vi "load_xml.vi"(8 "error in":errorcluster, 10 "child node in":refnum<k20>, 11 "DAQmx_pulse_out (in)":refnum<class "DAQmx_DO.lvclass">) -> (0 "error out":errorcluster, 2 "child node out":refnum<k20>, 3 "DAQmx_pulse_out":refnum<class "DAQmx_DO.lvclass">)   [LabVIEW 2014, in "DAQmx_DO.lvclass"]
doc: "Loads DAQmx pulse output settings from xml. Expected format:\n\n<EnableDAQmxPulses>%b</EnableDAQmxPulses>\n<ResourceName>%s</ResourceName>\n<ClockRate>%f</ClockRate>\n<unitsPerSecond>%f</unitsPerSecond>\n<StartTrigger.WaitForStartTrigger>%b</StartTrigger.WaitForStartTrigger>\n<StartTrigger.source>%s</StartTrigger.source>\n<StartTrigger.edge>%s</StartTrigger.edge>\n<TimingSequenceControl columns=\"Description, Active?, Idle State,Off 0,On 0,Off 1,On 1,etc.\">\n<channel>%s</channel>\n</TimingSequenceControl>\n\nMTL 2013 Jan 1"
uses:
  DAQmx_DO.lvclass
  DAQmx_DO.lvclass/DAQmx_DO.ctl
  Globals.vi
  <vilib>/xml/Close Reference(Node).vi
  <resource>/objmgr/DOMUserDefRef.rc
  <vilib>/xml/NI_XML.lvlib
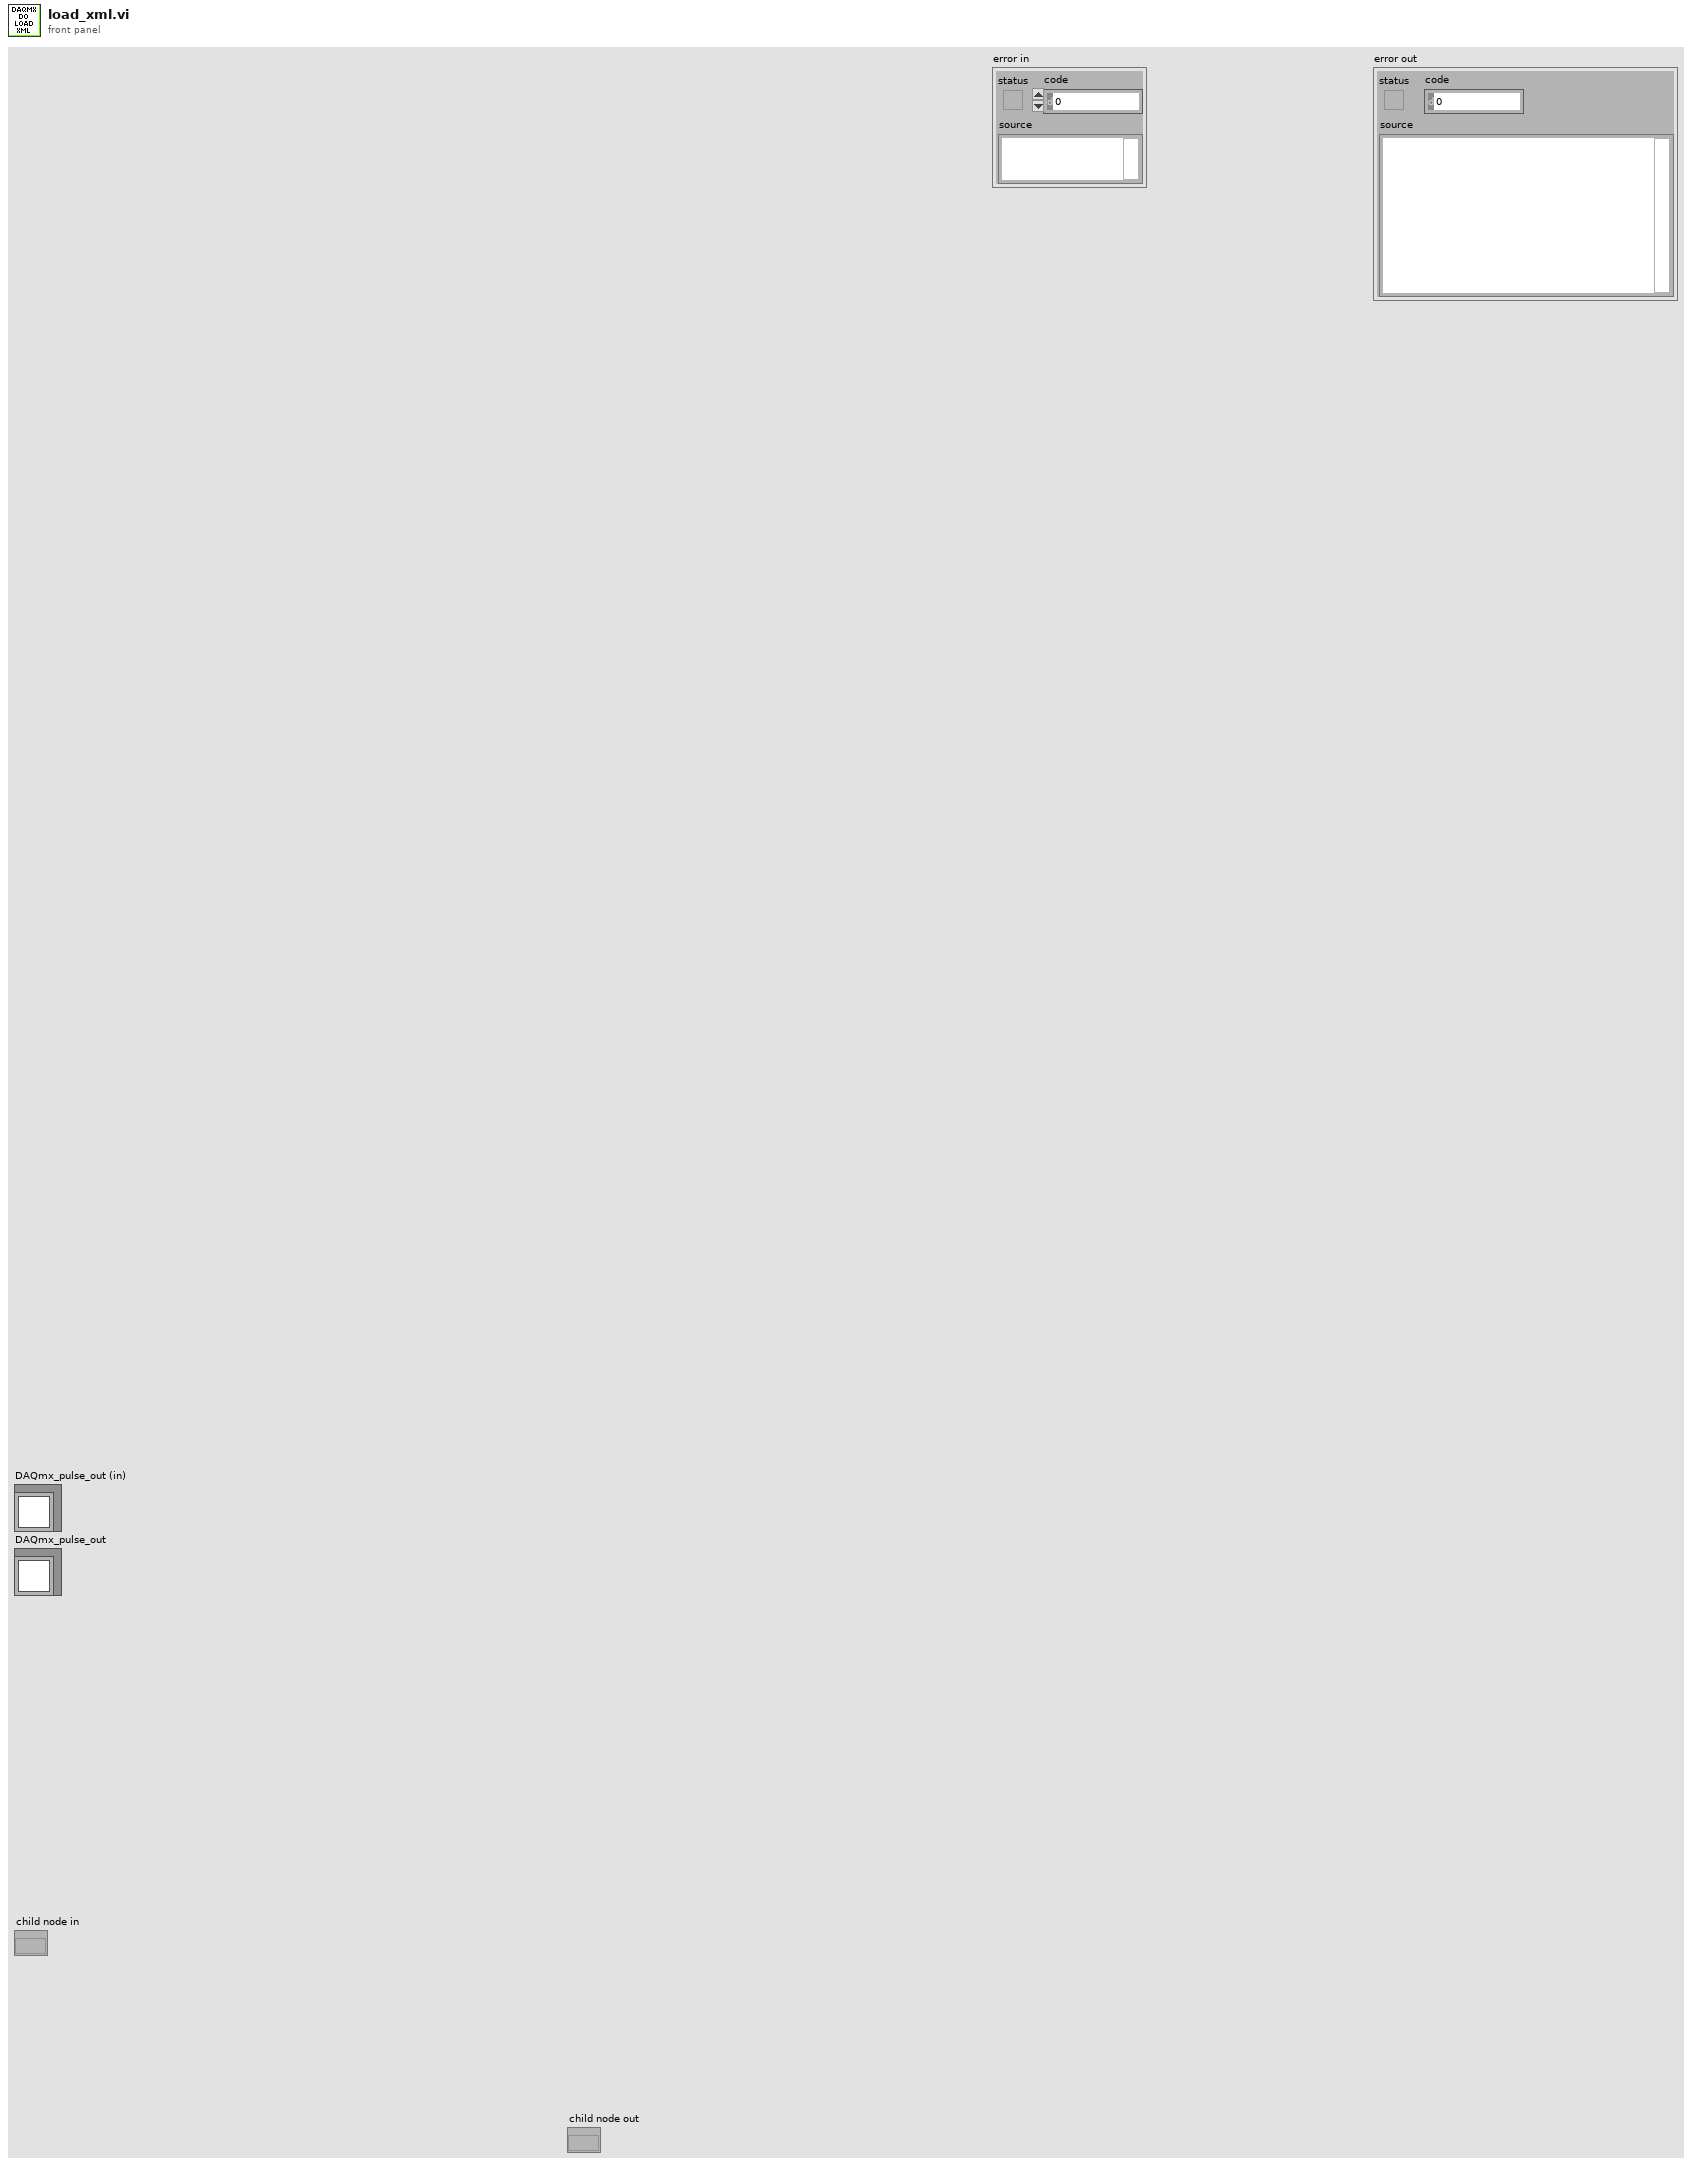
[diagram p1: front panel]
types:
  T1 = typedef "DAQmx_DO.lvclass/settings.ctl" = cluster{"Enable DAQmx Pulses":bool, "DAQmx Physical Channels":tag, "Clock Rate":dbl, "units/sec (ms=1000)":dbl, "Start Trigger":cluster{"Wait for start trigger?":bool, "source":tag, "edge":i32}, "waveform":T2}
  T2 = typedef "HSDIO.lvclass/waveform.ctl" = cluster{"name":string, "transitions":u32[], "states":u8[][]}
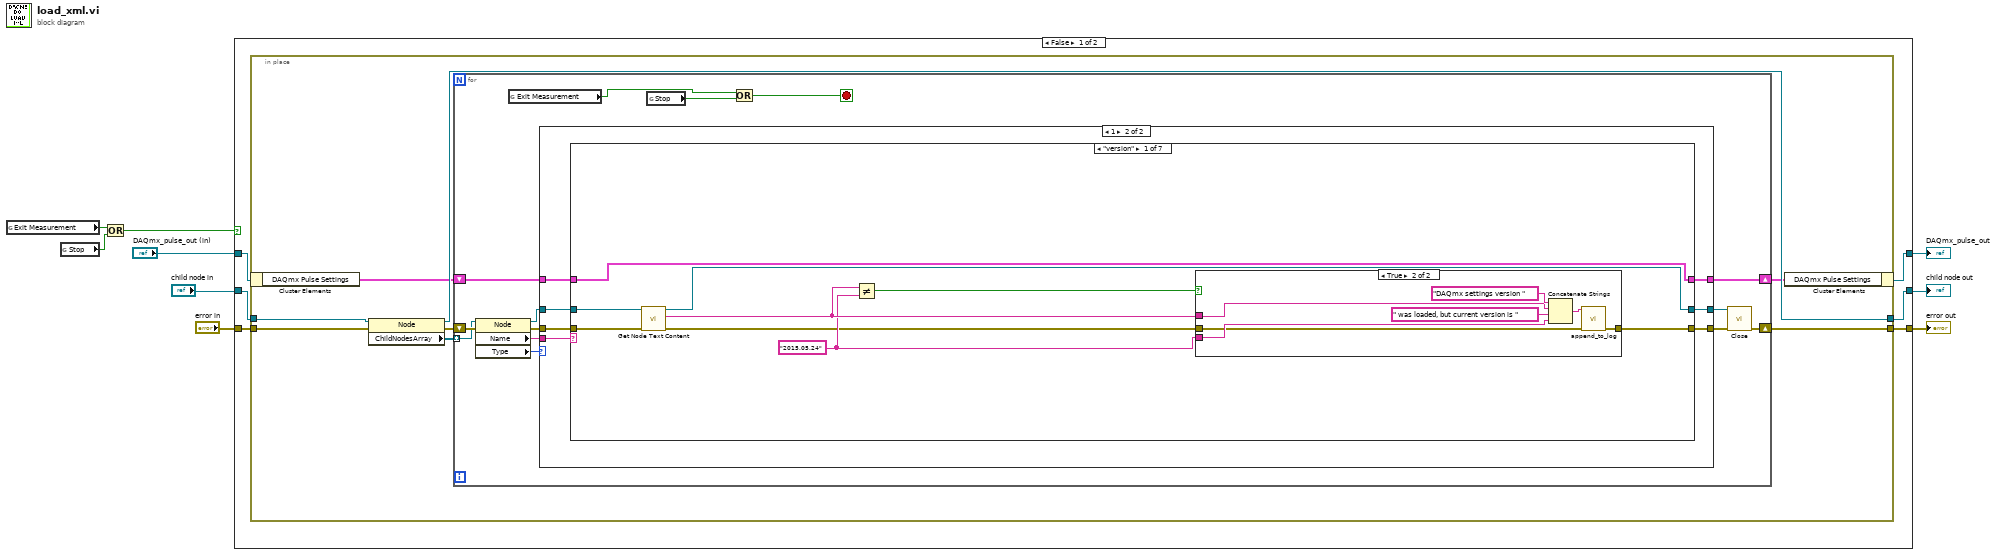
[diagram p0: block diagram]
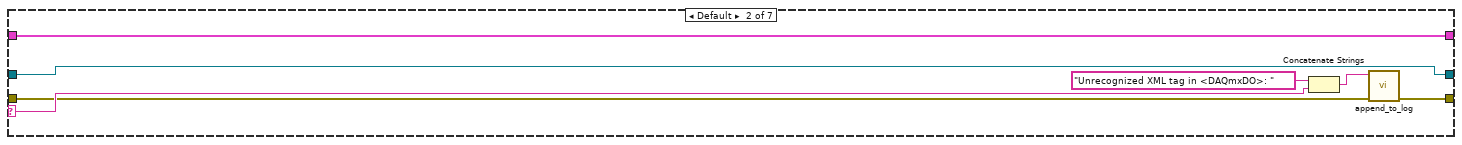
[diagram p4: hidden frame]
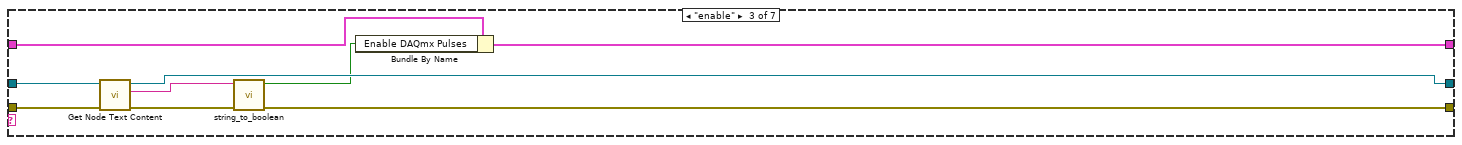
[diagram p5: hidden frame]
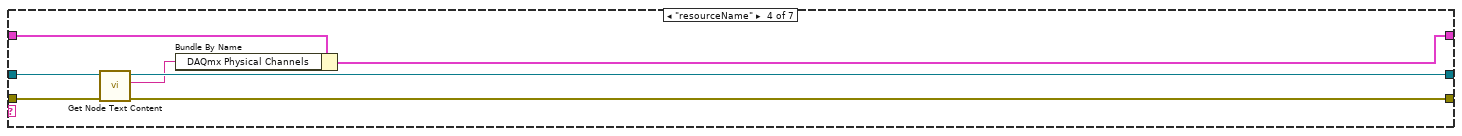
[diagram p6: hidden frame]
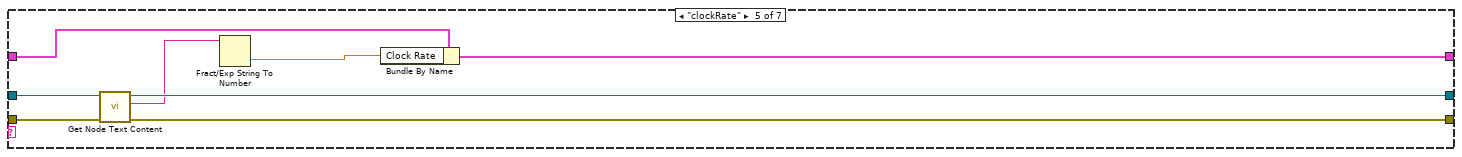
[diagram p7: hidden frame]
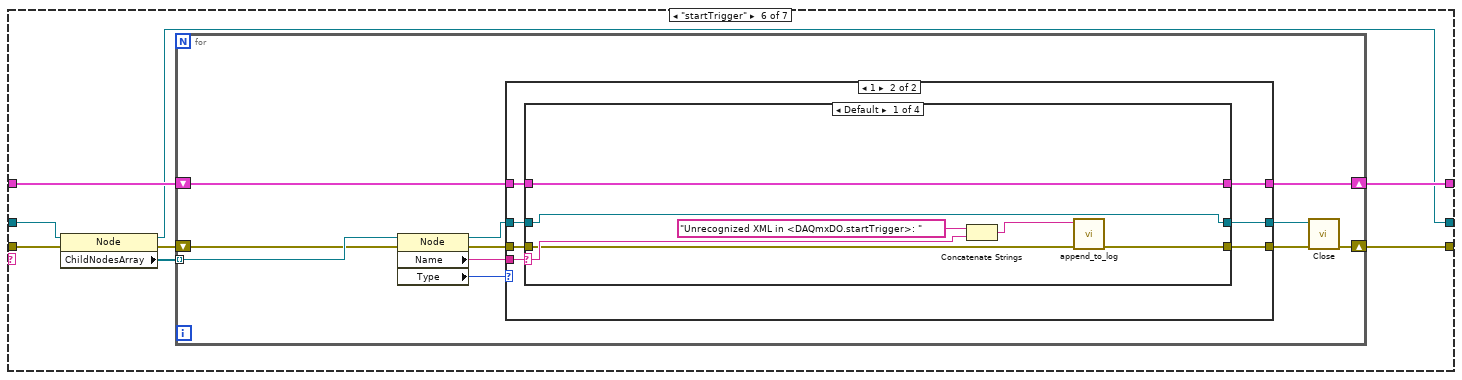
[diagram p8: hidden frame]
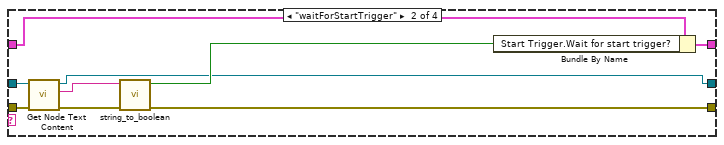
[diagram p10: hidden frame]
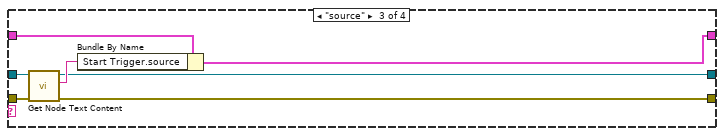
[diagram p11: hidden frame]
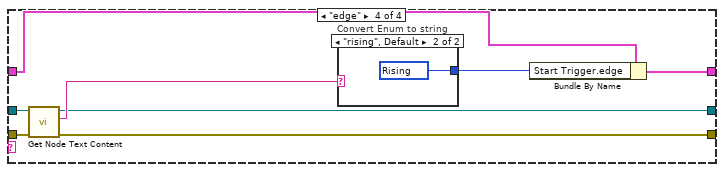
[diagram p12: hidden frame]
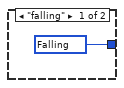
[diagram p13: hidden frame]
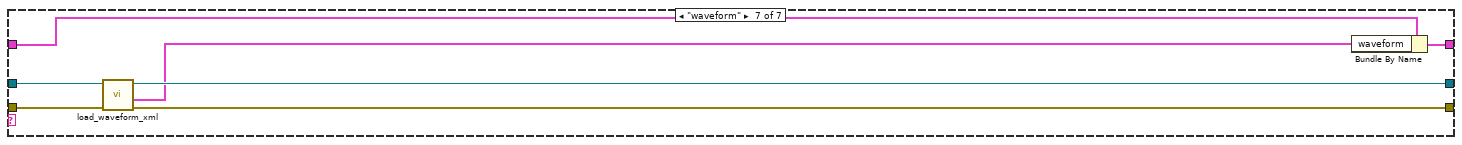
[diagram p14: hidden frame]
diagram:
  n1 = global read "Globals.vi" "Exit Measurement"() -> (w8:bool)
  n2 = global read "Globals.vi" "Stop"() -> (w9:bool)
  n3 = Or(x=w8, y=w9) -> (x .or. y?=w7:bool)
  n4 = case shown="False" w7 {
    tunnel: "DAQmx_pulse_out (in)" -> [w15 w167]
    tunnel: [w14 w167] -> w5
    tunnel: "error in" -> [w13 w166]
    tunnel: [w12 w166] -> w3
    tunnel: "child node in" -> [w11 w165]
    tunnel: [w10 w165] -> w1
    frame False {
      n5 = in-place {
        in-place-border: w13 -> [w21]
        in-place-border: [w20] -> w12
        in-place-border: w11 -> [w19]
        in-place-border: [w18] -> w10
        n6 = in-place-cluster #1(w15) -> ("DAQmx Pulse Settings"=w17:T1)
        n7 = property class="Node"(reference=w19, error in=w21) -> (reference out=w18:refnum<k20>, error out=w22:errorcluster, "ChildNodesArray"=w23:refnum<k20>[])
        n8 = for {
          tunnel: w23 -> [w28] mode=indexing
          shift-right: [w34] -> w16
          shift-left: w17 -> [w35]
          shift-right: [w31] -> w20
          shift-left: w22 -> [w29]
          stop <- w25 stop-if-true
          n9 = property class="Node"(reference=w28, error in=w29) -> (reference out=w36:refnum<k20>, error out=w32:errorcluster, "Name"=w37:string, "Type"=w24:i32)
          n10 = global read "Globals.vi" "Exit Measurement"() -> (w26:bool)
          n11 = case shown="1" w24 {
            tunnel: w37 -> [_ w47]
            tunnel: w36 -> [w39 w46]
            tunnel: w35 -> [w38 w45]
            tunnel: [w38 w44] -> w34
            tunnel: [w39 w43] -> w33
            tunnel: w32 -> [w40 w42]
            tunnel: [w40 w41] -> w30
            frame 0, Default {
            }
            frame 1 {
              n12 = case shown="\"version\"" w47 {
                selector: w47 -> [_ w67 _ _ _ _ _]
                tunnel: w46 -> [w51 w70 w79 w84 w92 w100 w162]
                tunnel: w45 -> [w49 w71 w77 w87 w95 w99 w164]
                tunnel: [w49 w71 w76 w86 w94 w97 w163] -> w44
                tunnel: [w50 w70 w80 w85 w93 w96 w161] -> w43
                tunnel: w42 -> [w52 w66 w78 w83 w91 w101 w159]
                tunnel: [w48 w65 w72 w82 w90 w98 w160] -> w41
                frame "version" {
                  w54 = "2015.05.24" ("y")
                  n13 = call <vilib>:"Get Node Text Content.vi"("error in (no error)"=w52, "node in"=w51) -> ("error out"=w53:errorcluster, "node text"=w55:string, "node out"=w50:refnum<k20>)  [unwired: 7 in]
                  n14 = Not Equal?(x=w55, y=w54) -> (x != y?=w56:bool)
                  n15 = case shown="True" w56 {
                    tunnel: w55 -> [_ w63]
                    tunnel: w54 -> [_ w61]
                    tunnel: w53 -> [w57 w59]
                    tunnel: [w57 w58] -> w48
                    frame False {
                    }
                    frame True {
                      n16 = Concatenate Strings("DAQmx settings version " ("string"), w63, " was loaded, but current version is " ("string"), w61) -> (w60:string)
                      n17 = call "append_to_log.vi"("error in"=w59, "string"=w60) -> ("error out"=w58:errorcluster)  [unwired: 9 in]
                    }
                  }
                }
                frame Default {
                  n18 = Concatenate Strings("Unrecognized XML tag in <DAQmxDO>: " ("string"), w67) -> (w68:string)
                  n19 = call "append_to_log.vi"("error in"=w66, "string"=w68) -> ("error out"=w65:errorcluster)  [unwired: 9 in]
                }
                frame "enable" {
                  n20 = call <vilib>:"Get Node Text Content.vi"("error in (no error)"=w78, "node in"=w79) -> ("error out"=w73:errorcluster, "node text"=w75:string, "node out"=w80:refnum<k20>)  [unwired: 7 in]
                  n21 = call "string_to_boolean.vi"("error in"=w73, "string"=w75) -> ("error out"=w72:errorcluster, "boolean"=w74:bool)  [unwired: 8 in]
                  n22 = Bundle By Name(cluster=w77, "Enable DAQmx Pulses"=w74) -> (w76:T1)
                }
                frame "resourceName" {
                  n23 = call <vilib>:"Get Node Text Content.vi"("error in (no error)"=w83, "node in"=w84) -> ("error out"=w82:errorcluster, "node text"=w81:string, "node out"=w85:refnum<k20>)  [unwired: 7 in]
                  n24 = Bundle By Name(cluster=w87, "DAQmx Physical Channels"=w81) -> (w86:T1)
                }
                frame "clockRate" {
                  n25 = call <vilib>:"Get Node Text Content.vi"("error in (no error)"=w91, "node in"=w92) -> ("error out"=w90:errorcluster, "node text"=w89:string, "node out"=w93:refnum<k20>)  [unwired: 7 in]
                  n26 = Fract/Exp String To Number(string=w89) -> (number=w88:dbl)  [unwired: 3 in, 1 out]
                  n27 = Bundle By Name(cluster=w95, "Clock Rate"=w88) -> (w94:T1)
                }
                frame "startTrigger" {
                  n28 = property class="Node"(reference=w100, error in=w101) -> (reference out=w96:refnum<k20>, error out=w102:errorcluster, "ChildNodesArray"=w103:refnum<k20>[])
                  n29 = for {
                    tunnel: w103 -> [w114] mode=indexing
                    shift-right: [w106] -> w98
                    shift-left: w102 -> [w113]
                    shift-right: [w104] -> w97
                    shift-left: w99 -> [w105]
                    n30 = property class="Node"(reference=w114, error in=w113) -> (reference out=w110:refnum<k20>, error out=w109:errorcluster, "Name"=w111:string, "Type"=w112:i32)
                    n31 = case shown="1" w112 {
                      tunnel: w111 -> [_ w124]
                      tunnel: w110 -> [w116 w123]
                      tunnel: [w117 w119] -> w107
                      tunnel: w109 -> [w117 w120]
                      tunnel: [w116 w118] -> w108
                      tunnel: w105 -> [w115 w122]
                      tunnel: [w115 w121] -> w104
                      frame Default {
                      }
                      frame 1 {
                        n32 = case shown="Default" w124 {
                          selector: w124 -> [w127 _ _ _]
                          tunnel: w123 -> [w128 w135 w144 w154]
                          tunnel: w122 -> [w129 w137 w146 w151]
                          tunnel: [w129 w136 w145 w150] -> w121
                          tunnel: w120 -> [w126 w134 w142 w152]
                          tunnel: [w125 w133 w141 w149] -> w119
                          tunnel: [w128 w132 w143 w153] -> w118
                          frame Default {
                            n33 = Concatenate Strings("Unrecognized XML in <DAQmxDO.startTrigger>: " ("string"), w127) -> (w130:string)
                            n34 = call "append_to_log.vi"("error in"=w126, "string"=w130) -> ("error out"=w125:errorcluster)  [unwired: 9 in]
                          }
                          frame "waitForStartTrigger" {
                            n35 = call <vilib>:"Get Node Text Content.vi"("error in (no error)"=w134, "node in"=w135) -> ("error out"=w138:errorcluster, "node text"=w140:string, "node out"=w132:refnum<k20>)  [unwired: 7 in]
                            n36 = call "string_to_boolean.vi"("error in"=w138, "string"=w140) -> ("error out"=w133:errorcluster, "boolean"=w139:bool)  [unwired: 8 in]
                            n37 = Bundle By Name(cluster=w137, "Start Trigger.Wait for start trigger?"=w139) -> (w136:T1)
                          }
                          frame "source" {
                            n38 = call <vilib>:"Get Node Text Content.vi"("error in (no error)"=w142, "node in"=w144) -> ("error out"=w141:errorcluster, "node text"=w147:string, "node out"=w143:refnum<k20>)  [unwired: 7 in]
                            n39 = Bundle By Name(cluster=w146, "Start Trigger.source"=w147) -> (w145:T1)
                          }
                          frame "edge" {
                            n40 = call <vilib>:"Get Node Text Content.vi"("error in (no error)"=w152, "node in"=w154) -> ("error out"=w149:errorcluster, "node text"=w155:string, "node out"=w153:refnum<k20>)  [unwired: 7 in]
                            n41 = case "Convert Enum to string" shown="\"rising\", Default" w155 {
                              tunnel: [w156 w157] -> w148
                              frame "falling" {
                                w156 = 10171 items=["Rising"=10280, "Falling"=10171] ("edge")
                              }
                              frame "rising", Default {
                                w157 = 10280 items=["Rising"=10280, "Falling"=10171] ("edge")
                              }
                            }
                            n42 = Bundle By Name(cluster=w151, "Start Trigger.edge"=w148) -> (w150:T1)
                          }
                        }
                      }
                    }
                    n43 = call-poly <vilib>:"Close.vi"("error in (no error)"=w107, "node"=w108) -> ("error out"=w106:errorcluster)  [unwired: 7 in]
                  }
                }
                frame "waveform" {
                  n44 = call "load_waveform_xml.vi"("error (in)"=w159, "Node (in)"=w162) -> ("error"=w160:errorcluster, "Waveform prototype"=w158:T2, "Node"=w161:refnum<k20>)  [unwired: 7 in]
                  n45 = Bundle By Name(cluster=w164, "waveform"=w158) -> (w163:T1)
                }
              }
            }
          }
          n46 = global read "Globals.vi" "Stop"() -> (w27:bool)
          n47 = Or(x=w26, y=w27) -> (x .or. y?=w25:bool)
          n48 = call-poly <vilib>:"Close.vi"("error in (no error)"=w30, "node"=w33) -> ("error out"=w31:errorcluster)  [unwired: 7 in]
        }
        n49 = in-place-cluster #1("DAQmx Pulse Settings"=w16) -> (w14:refnum<class "DAQmx_DO.lvclass">)
      }
    }
    frame True {
    }
  }
  "DAQmx_pulse_out" <- w5
  "error out" <- w3
  "child node out" <- w1
